vi "Powspec.vi"(0 "Emg input":dbl[](array[numeric]) format="%.2f", 1 "Sample rate":sgl=1024.0 format="%.2f") -> (2 "Median Power Frequency":dbl format="%.2f", 3 "Mean Power Frequency":dbl format="%.2f", 4 "Spectrum Plot":cluster{dbl, "df":dbl, dbl[]}(graph)={0.0, "df"=0.5, []}, 5 "Estimated Peak Frequency":dbl format="%.2f", 6 "Estimated Peak Power":dbl format="%.2f", 7 "Spectrum Unit":string="Vrms^2/Hz")   [LabVIEW 2011]
doc: "This example shows how to construct a simple Spectrum Analyzer example using the EASY I/O DAQ VIs and the MEASUREMENT VIs. This example acquires a waveform, windows it, computes the autopower spectrum and the power and frequency of the peak frequency component. The power spectrum is graphed in the desired units."
uses:
  <vilib>/Analysis/NI_AALPro.lvlib
  <vilib>/Analysis/0measdsp.llb/Scaled Time Domain Window (DBL).vi
panel:
  in  "Display Unit":i32(ring)=6 items=["Vrms", "Vpk", "Vrms^2", "Vpk^2", "Vrms/rtHz", "Vpk/rtHz", "Vrms^2/Hz", "Vpk^2/Hz"]
  in  "Log/Linear":enum16{"Linear", "dB", "dBm"}(ring)
  in  "Window":i32(ring)=2 items=["None (Uniform)", "Hann", "Hamming", "Blackman-Harris", "Exact Blackman", "Blackman", "Flat Top", "4 Term B-Harris", "7 Term B-Harris"]
  # "Hz"
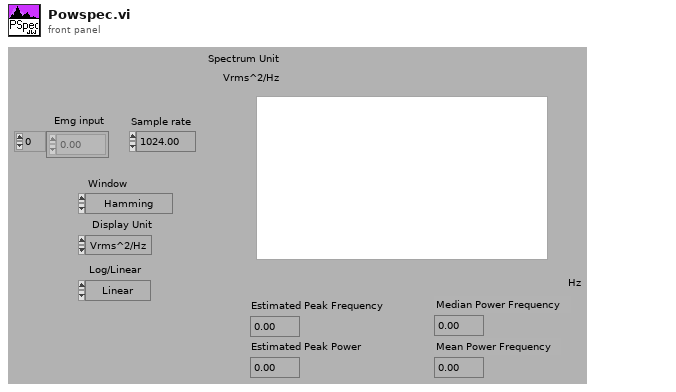
[diagram p1: front panel]
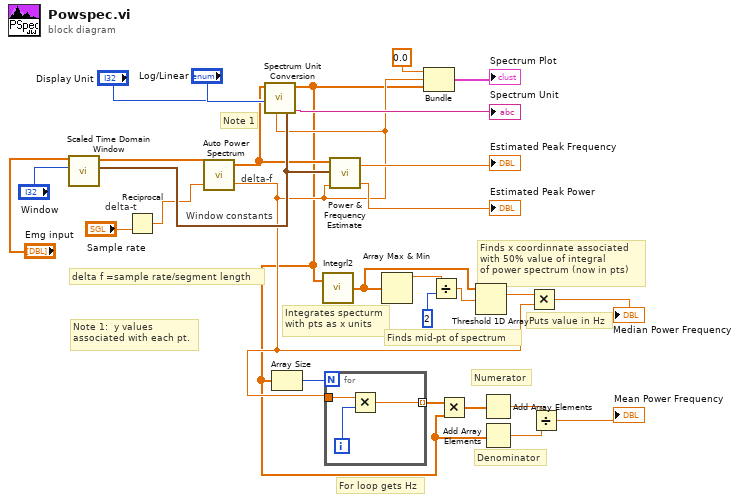
[diagram p0: block diagram]
diagram:
  # "Denominator"
  # "For loop gets Hz"
  # "Numerator"
  # "Puts value in Hz"
  # "Finds mid-pt of spectrum"
  # "Finds x coordinnate associated\nwith 50% value of integral\nof power spectrum (now in pts)"
  # "Integrates specturm\nwith pts as x units"
  # "Note 1"
  # "Note 1:  y values\nassociated with each pt."
  # "delta f =sample rate/segment length"
  # "Window constants"
  # "delta-f"
  # "delta-t"
  n1 = call-poly <vilib>:"Scaled Time Domain Window.vi"("window"="Window", "X"="Emg input") -> ("window properties"=w25:cluster{"eq noise BW":dbl, "coherent gain":dbl}, "Windowed X"=w27:dbl[])  [unwired: 7 in, 1 out]
  n2 = Reciprocal(x="Sample rate") -> (1/x=w21:sgl)
  n3 = call <vilib>:"Auto Power Spectrum.vi"("dt"=w21, "Signal (V)"=w27) -> ("df"=w6:dbl, "Power Spectrum (V^2 rms)"=w20:dbl[])
  n4 = call <vilib>:"Spectrum Unit Conversion.vi"("window constants"=w25, "df"=w6, "display unit"="Display Unit", "log/linear"="Log/Linear", "Spectrum in"=w20) -> ("spectrum unit"=→"Spectrum Unit":string, "Spectrum out"=w4:dbl[])  [unwired: 5 in]
  n5 = Array Size(array=w4) -> (size(s)=w8:i32)
  n6 = call "Integrl2.vi"("Input Array"=w4) -> ("Output Array (Integral)"=w11:dbl[])  [unwired: 1 in]
  n7 = for {
    N: w8 -> [_]
    tunnel: w6 -> [w30]
    tunnel: [w29] -> w7 mode=indexing
    i -> [w31]
    n8 = Multiply(x=w30, y=w31) -> (x*y=w29:dbl)
  }
  n9 = call <vilib>:"Power & Frequency Estimate.vi"("df"=w6, "window constants"=w25, "Power Spectrum (V^2 rms)"=w20) -> ("est power peak"=→"Estimated Peak Power":dbl, "est frequency peak"=→"Estimated Peak Frequency":dbl)  [unwired: 3 in]
  n10 = Array Max & Min(array=w11) -> (max value=w14:dbl)  [unwired: 3 out]
  n11 = Bundle(0.0, "df"=w6, "Spectrum out"=w4) -> (→"Spectrum Plot":cluster{dbl, "df":dbl, "Spectrum out":dbl[]})  [unwired: 1 in]
  n12 = Divide(x=w14, y=2) -> (x/y=w12:dbl)
  n13 = Multiply(x=w7, y=w4) -> (x*y=w5:dbl[])
  n14 = Threshold 1D Array(2:w12, 3:w11) -> (0:w10:dbl)  [unwired: 1 in]
  n15 = Add Array Elements(numeric array=w5) -> (sum=w3:dbl)
  n16 = Add Array Elements(numeric array=w4) -> (sum=w2:dbl)
  n17 = Multiply(x=w10, y=w6) -> (x*y=→"Median Power Frequency":dbl)
  n18 = Divide(x=w3, y=w2) -> (x/y=→"Mean Power Frequency":dbl)
